vi "test.formatVariantIntoString.vi"() -> ()   [LabVIEW 2017]
panel:
  out "Data 2":string
  out "Data":string
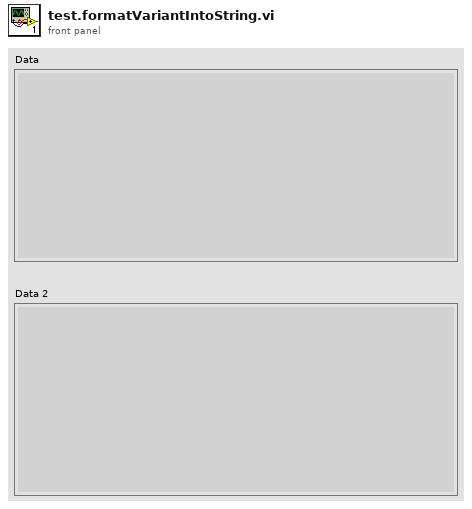
[diagram p1: front panel]
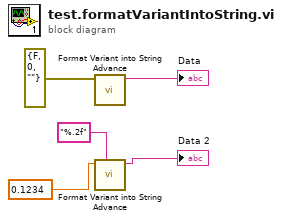
[diagram p0: block diagram]
diagram:
  n1 = call "Format Variant into String Advance.vi"("Variant"=errorcluster {"status"=FALSE, "code"=0, "source"=""} ("error in (no error)")) -> ("Data"=→"Data":string)  [unwired: 8 in, 2 out]
  n2 = call "Format Variant into String Advance.vi"("Format String"="%.2f", "Variant"=0.1234 ("code")) -> ("Data"=→"Data 2":string)  [unwired: 7 in, 2 out]
